vi "LVClass_WavefrontCorrector Set Actuator Preferences.vi"(0 "WavefrontCorrector in":refnum<class "WavefrontCorrector.lvclass">, 5 "Index of actuator":i32, 7 "Wavefront Corrector state":T1, 11 "error in (no error)":errorcluster) -> (4 "WavefrontCorrector out":refnum<class "WavefrontCorrector.lvclass">, 15 "error out":errorcluster)   [LabVIEW 2020, in "WavefrontCorrector.lvclass"]
doc: "Set preferences of actuator.\n\n<B>correctorIn</B> : WavefrontCorrector object.\n<B>correctorOut</B> : WavefrontCorrector object.\n<B>actuator_index</B> : Index of the actuator.\n<B>min</B> : WavefrontCorrector actuator preferences : lowest command value.\n<B>max</B> : WavefrontCorrector actuator preferences : highest command value.\n<B>validity</B> : WavefrontCorrector actuator preferences : status.\n<B>fixed_value</B> : WavefrontCorrector actuator preferences : fixed positions."
uses:
  WavefrontCorrector.lvclass
  Wavefront Corrector states - ONE.ctl
  WavefrontCorrector.lvclass/WavefrontCorrector.ctl
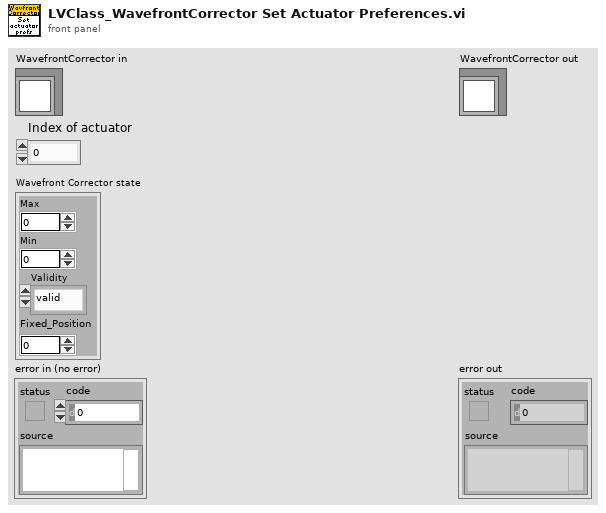
[diagram p1: front panel]
types:
  T1 = typedef "Wavefront Corrector states - ONE.ctl" = cluster{"Max":sgl, "Min":sgl, "Validity":enum16{"valid", "fixed", "invalid"}, "Fixed_Position":sgl}
  T2 = typedef "ClassID.ctl" = i64
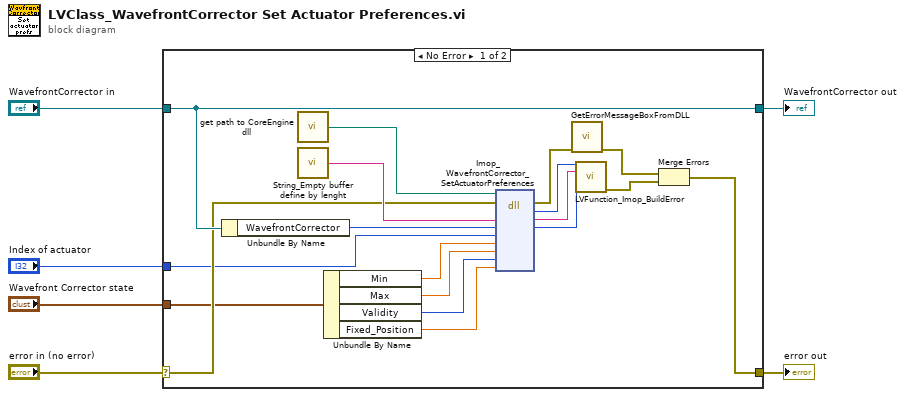
[diagram p0: block diagram]
diagram:
  n1 = case shown="No Error" "error in (no error)" {
    selector: "error in (no error)" -> [w15 w26]
    tunnel: [w14 w26] -> w5
    tunnel: [w16 w25] -> w3
    tunnel: "WavefrontCorrector in" -> [w16 w25]
    tunnel: "Wavefront Corrector state" -> [w13 _]
    tunnel: "Index of actuator" -> [w8 _]
    frame No Error {
      n2 = Unbundle By Name(w16) -> ("WavefrontCorrector"=w22:T2)
      n3 = call "get path to CoreEngine dll.vi"() -> ("path to wavekit library"=w24:path)  [unwired: 14 in, 1 out]
      n4 = call "String_Empty buffer define by lenght.vi"() -> ("Empty buffer"=w23:string)  [unwired: 1 in]
      n5 = Unbundle By Name(w13) -> ("Min"=w12:sgl, "Max"=w11:sgl, "Validity"=w10:enum16{"valid", "fixed", "invalid"}, "Fixed_Position"=w9:sgl)
      n6 = dll-call lib="D:/FLE/0.Code/CoreEngine4_Suite/LV2011_interface/DLLs/c_interface_vc100.dll" fn="Imop_WavefrontCorrector_SetActuatorPreferences"(path in=w24, error in=w15, "Message"=w23, "Wavefront Corrector"=w22, "Index of actuator"=w8, "Min"=w12, "Max"=w11, "Validity"=w10, "Fixed_positions"=w9) -> (error out=w21:errorcluster, "return type"=w19:i32, "Message"=w18:string, "Wavefront Corrector"=w7:i64)  [unwired: 6 in, 1 out]
      n7 = call "GetErrorMessageBoxFromDLL.vi"("error IN"=w21) -> ("error OUT"=w20:errorcluster)  [unwired: 10 in]
      n8 = call "LVFunction_Imop_BuildError.vi"("code"=w19, "String to Prepend to source (\"\")"=w18, "Adresse"=w7) -> ("error out"=w17:errorcluster)  [unwired: 12 in]
      n9 = Merge Errors(w20, w17) -> (w14:errorcluster)
    }
    frame Error {
    }
  }
  "error out" <- w5
  "WavefrontCorrector out" <- w3
